vi "sendValveSignal-v03.vi"(0 "daq_do":tag="Dev1/ai0:1", 1 "Set Status":bool, 3 "Valve1?":bool, 5 "ChangeToValve":u16, 9 "CurrentValve":u16, 11 "controls array in":refnum<vi>[](array[refnum]), 12 "time to wait for solution change (min)":dbl=2.5 min=0.0 step=0.01, 13 "valve Time Cluster":T1) -> (6 "ValveSetTo":u16, 10 "valve changed?":bool, 14 "additional time to wait (min)":dbl=2.5 min=0.0 step=0.01, 15 "control array out":refnum<vi>[](array[refnum]))   [LabVIEW 2019]
uses:
  <vilib>/DAQmx/write.llb/DAQmx Write (Digital 1D Bool NChan 1Samp 1Line).vi
  <vilib>/DAQmx/miscellaneous.llb/DAQmx Fill In Error Info.vi
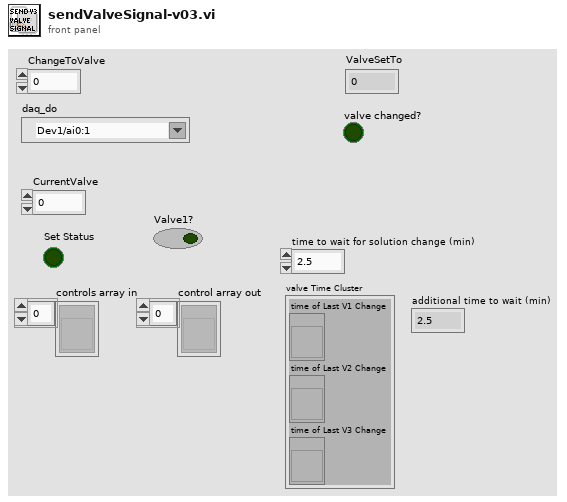
[diagram p1: front panel]
types:
  T1 = cluster{"time of Last V1 Change":refnum<vi>, "time of Last V2 Change":refnum<vi>, "time of Last V3 Change":refnum<vi>}
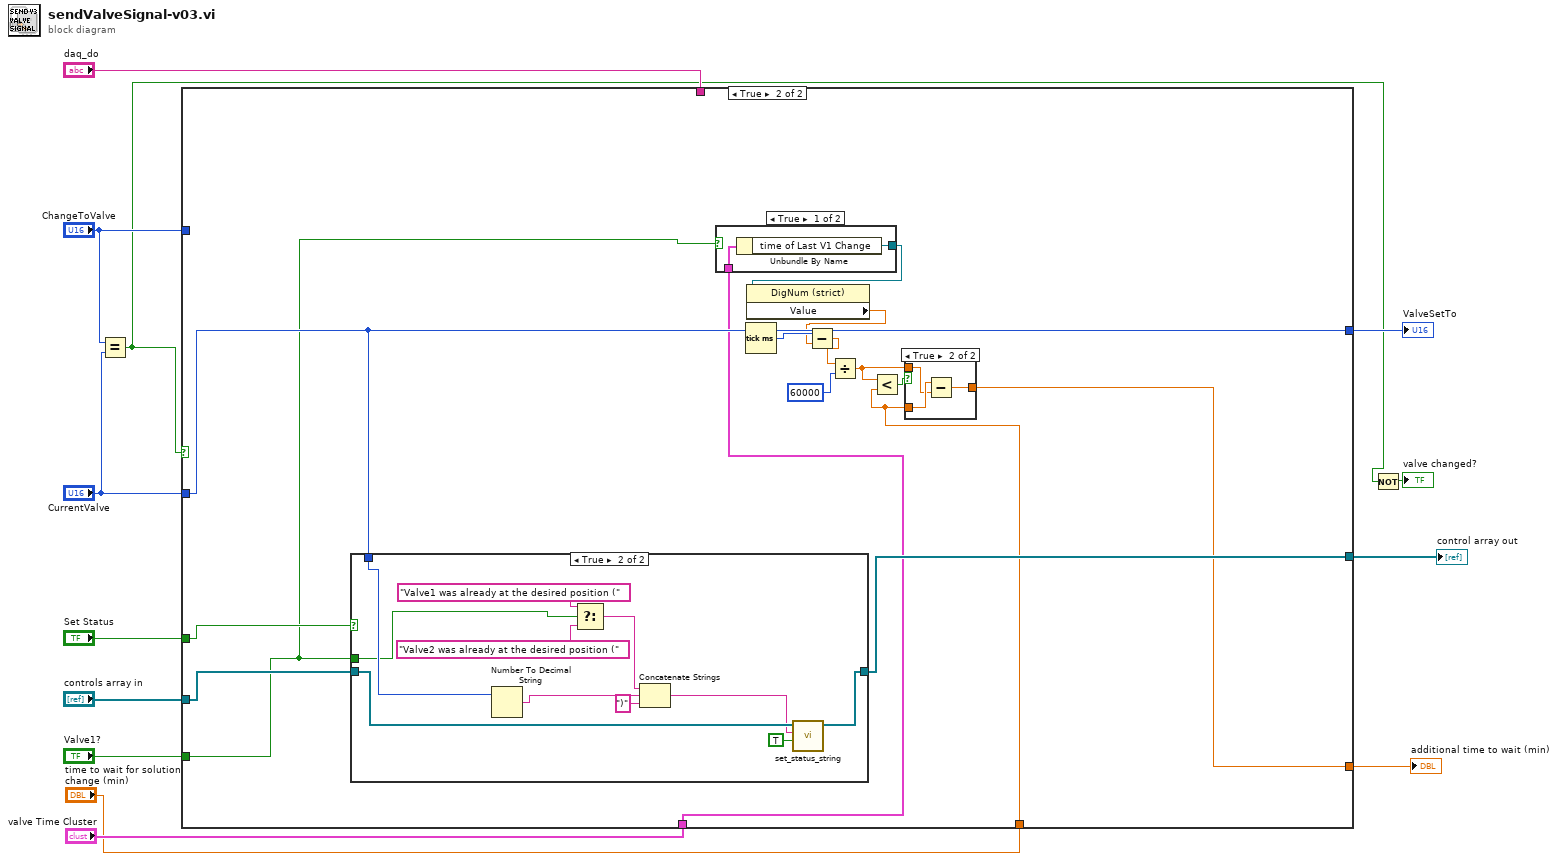
[diagram p0: block diagram]
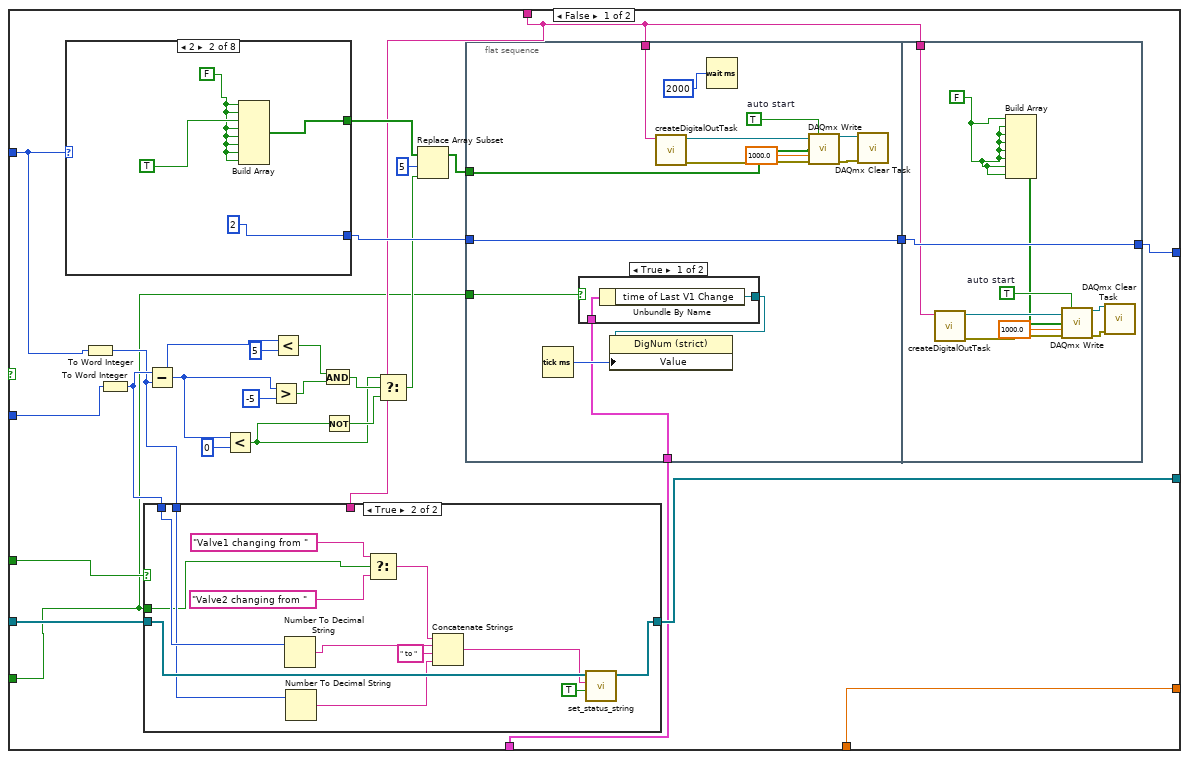
[diagram p2: hidden frame]
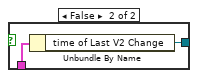
[diagram p4: hidden frame]
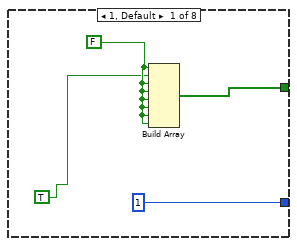
[diagram p5: hidden frame]
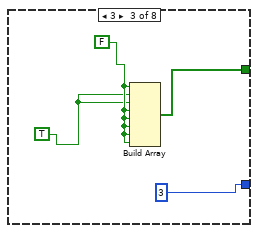
[diagram p6: hidden frame]
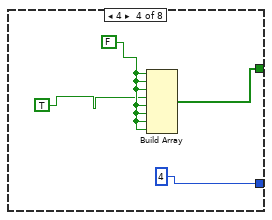
[diagram p7: hidden frame]
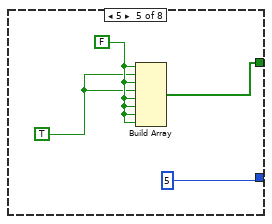
[diagram p8: hidden frame]
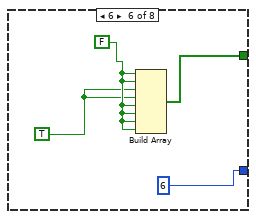
[diagram p9: hidden frame]
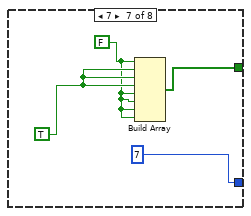
[diagram p10: hidden frame]
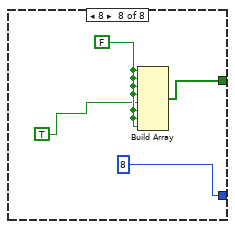
[diagram p11: hidden frame]
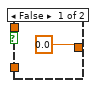
[diagram p12: hidden frame]
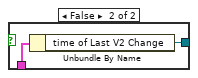
[diagram p13: hidden frame]
diagram:
  n1 = Equal?(x="ChangeToValve", y="CurrentValve") -> (x = y?=w4:bool)
  n2 = case shown="True" w4 {
    tunnel: [w38 w127] -> w13
    tunnel: "Set Status" -> [w24 w129]
    tunnel: "controls array in" -> [w23 w128]
    tunnel: [w22 w126] -> w10
    tunnel: "daq_do" -> [w17 _]
    tunnel: "Valve1?" -> [w14 w119]
    tunnel: "ChangeToValve" -> [w19 _]
    tunnel: "CurrentValve" -> [w18 w127]
    tunnel: [w16 w117] -> w3
    tunnel: "valve Time Cluster" -> [w15 w120]
    tunnel: "time to wait for solution change (min)" -> [w16 w118]
    frame False {
      n3 = case shown="2" w19 {
        tunnel: [w86 w90 w94 w98 w102 w106 w110 w114] -> w28
        tunnel: [u16 1 u16 2 u16 3 u16 4 u16 5 u16 6 u16 7 u16 8] -> w39
        frame 1, Default {
          w84 = FALSE
          n4 = Build Array(w84, TRUE, w84, w84, w84, w84, w84, w84) -> (w86:bool[])
        }
        frame 2 {
          w87 = FALSE
          n5 = Build Array(w87, w87, TRUE, w87, w87, w87, w87, w87) -> (w90:bool[])
        }
        frame 3 {
          w92 = FALSE
          w91 = TRUE
          n6 = Build Array(w92, w91, w91, w92, w92, w92, w92, w92) -> (w94:bool[])
        }
        frame 4 {
          w96 = FALSE
          n7 = Build Array(w96, w96, w96, TRUE, w96, w96, w96, w96) -> (w98:bool[])
        }
        frame 5 {
          w100 = FALSE
          w99 = TRUE
          n8 = Build Array(w100, w99, w100, w99, w100, w100, w100, w100) -> (w102:bool[])
        }
        frame 6 {
          w104 = FALSE
          w103 = TRUE
          n9 = Build Array(w104, w104, w103, w103, w104, w104, w104, w104) -> (w106:bool[])
        }
        frame 7 {
          w107 = FALSE
          w108 = TRUE
          n10 = Build Array(w107, w108, w108, w108, w107, w107, w107, w107) -> (w110:bool[])
        }
        frame 8 {
          w112 = FALSE
          n11 = Build Array(w112, w112, w112, w112, TRUE, w112, w112, w112) -> (w114:bool[])
        }
      }
      n12 = To Word Integer(number=w19) -> (16bit integer=w20:i16)
      n13 = To Word Integer(number=w18) -> (16bit integer=w21:i16)
      n14 = case shown="True" w24 {
        tunnel: [w41 w52] -> w22
        tunnel: w23 -> [w41 w53]
        tunnel: w17 -> [_ _]
        tunnel: w21 -> [_ w48]
        tunnel: w20 -> [_ w45]
        tunnel: w14 -> [_ w42]
        frame False {
        }
        frame True {
          n15 = Number To Decimal String(number=w48) -> (decimal integer string=w47:string)  [unwired: 1 in]
          n16 = Number To Decimal String(number=w45) -> (decimal integer string=w44:string)  [unwired: 1 in]
          n17 = Select(t="Valve1 changing from ", s=w42, f="Valve2 changing from ") -> (s? t:f=w49:string)
          n18 = Concatenate Strings(w49, w47, " to " ("string"), w44) -> (w43:string)
          n19 = call "set_status_string.vi"("new line?"=TRUE, "status string in"=w43, "controls array"=w53) -> ("controls array out"=w52:refnum<vi>[])  [unwired: 7 in, 1 out]
        }
      }
      n20 = Subtract(x=w21, y=w20) -> (x-y=w35:i16)
      n21 = Less?(x=w35, y=i16 0) -> (x < y?=w29:bool)
      n22 = Greater?(x=w35, y=i16 -5) -> (0:w32:bool)
      n23 = Less?(x=w35, y=i16 5) -> (x < y?=w33:bool)
      n24 = And(x=w33, y=w32) -> (x .and. y?=w31:bool)
      n25 = Not(x=w29) -> (.not. x?=w30:bool)
      n26 = Select(t=w29, s=w31, f=w30) -> (s? t:f=w25:bool)
      n27 = Replace Array Subset(array=w28, new element=w25, index=5) -> (w27:bool[])
      n28 = flat-sequence {
        tunnel: w17 -> [w63]
        tunnel: w27 -> [w64]
        tunnel: w39 -> [w62]
        tunnel: [w62] -> w40
        tunnel: w15 -> [w56]
        tunnel: w14 -> [w55]
        tunnel: w40 -> [w82]
        tunnel: [w82] -> w38
        tunnel: w17 -> [w77]
        frame #0 {
          w67 = TRUE  # auto start
          n29 = Tick Count (ms)() -> (millisecond timer value=w57:u32)
          n30 = case shown="True" w55 {
            tunnel: w56 -> [w70 w72]
            tunnel: [w69 w71] -> w58
            frame True {
              n31 = Unbundle By Name(w70) -> ("time of Last V1 Change"=w69:refnum<vi>)
            }
            frame False {
              n32 = Unbundle By Name(w72) -> ("time of Last V2 Change"=w71:refnum<vi>)
            }
          }
          n33 = property class="DigNum (strict)"(reference=w58, "Value"=w57) -> ()  [unwired: 1 in, 2 out]
          n34 = call "createDigitalOutTask.vi"("daq_do"=w63) -> ("error out"=w65:errorcluster, "task out"=w66:refnum<k21>)  [unwired: 9 in]
          n35 = Wait (ms)(milliseconds to wait=u32 2000) -> ()  [unwired: 1 out]
          n36 = call-poly <vilib>:"DAQmx Write.vi"("task/channels in"=w66, "auto start"=w67, "data"=w64, "timeout"=1000.0, "error in"=w65) -> ("task out"=w60:refnum<k21>, "error out"=w59:errorcluster)  [unwired: 8 in, 1 out]
          n37 = call <vilib>:"DAQmx Clear Task.vi"("task in"=w60, "error in"=w59) -> ()  [unwired: 13 in, 1 out]
        }
        frame #1 {
          w75 = FALSE
          w81 = TRUE  # auto start
          n38 = call "createDigitalOutTask.vi"("daq_do"=w77) -> ("error out"=w79:errorcluster, "task out"=w80:refnum<k21>)  [unwired: 9 in]
          n39 = Build Array(w75, w75, w75, w75, w75, w75, w75, w75) -> (w78:bool[])
          n40 = call-poly <vilib>:"DAQmx Write.vi"("task/channels in"=w80, "auto start"=w81, "data"=w78, "timeout"=1000.0, "error in"=w79) -> ("task out"=w74:refnum<k21>, "error out"=w73:errorcluster)  [unwired: 8 in, 1 out]
          n41 = call <vilib>:"DAQmx Clear Task.vi"("task in"=w74, "error in"=w73) -> ()  [unwired: 13 in, 1 out]
        }
      }
    }
    frame True {
      n42 = case shown="True" w129 {
        tunnel: [w138 w147] -> w126
        tunnel: w128 -> [w138 w148]
        tunnel: w127 -> [_ w143]
        tunnel: w119 -> [_ w139]
        frame False {
        }
        frame True {
          n43 = Number To Decimal String(number=w143) -> (decimal integer string=w142:string)  [unwired: 1 in]
          n44 = Select(t="Valve1 was already at the desired position (", s=w139, f="Valve2 was already at the desired position (") -> (s? t:f=w144:string)
          n45 = Concatenate Strings(w144, w142, ")" ("string")) -> (w140:string)
          n46 = call "set_status_string.vi"("new line?"=TRUE, "status string in"=w140, "controls array"=w148) -> ("controls array out"=w147:refnum<vi>[])  [unwired: 7 in, 1 out]
        }
      }
      n47 = case shown="True" w119 {
        tunnel: w120 -> [w135 w137]
        tunnel: [w134 w136] -> w121
        frame True {
          n48 = Unbundle By Name(w135) -> ("time of Last V1 Change"=w134:refnum<vi>)
        }
        frame False {
          n49 = Unbundle By Name(w137) -> ("time of Last V2 Change"=w136:refnum<vi>)
        }
      }
      n50 = Tick Count (ms)() -> (millisecond timer value=w116:u32)
      n51 = property class="DigNum (strict)"(reference=w121) -> ("Value"=w115:dbl)  [unwired: 1 in, 2 out]
      n52 = Subtract(x=w116, y=w115) -> (x-y=w123:dbl)
      n53 = Divide(x=w123, y=u32 60000) -> (x/y=w125:dbl)
      n54 = Less?(x=w125, y=w118) -> (x < y?=w124:bool)
      n55 = case shown="True" w124 {
        tunnel: w118 -> [_ w133]
        tunnel: w125 -> [_ w132]
        tunnel: [0.0 ("additional time to wait (min)") w131] -> w117
        frame False {
        }
        frame True {
          n56 = Subtract(x=w133, y=w132) -> (x-y=w131:dbl)
        }
      }
    }
  }
  "ValveSetTo" <- w13
  "control array out" <- w10
  "additional time to wait (min)" <- w3
  n57 = Not(x=w4) -> (.not. x?=→"valve changed?":bool)
